vi "Write Service.vi"(8 "error in (no error)":errorcluster, 10 "Service":string, 11 "AWS Core in":refnum<class "NI_AWS_Core.lvclass">) -> (0 "error out":errorcluster, 3 "AWS Core out":refnum<class "NI_AWS_Core.lvclass">)   [LabVIEW 2015, in "NI_AWS_Core.lvclass"]
uses:
  NI_AWS_Core.lvclass
  NI_AWS_Core.lvclass/NI_AWS_Core.ctl
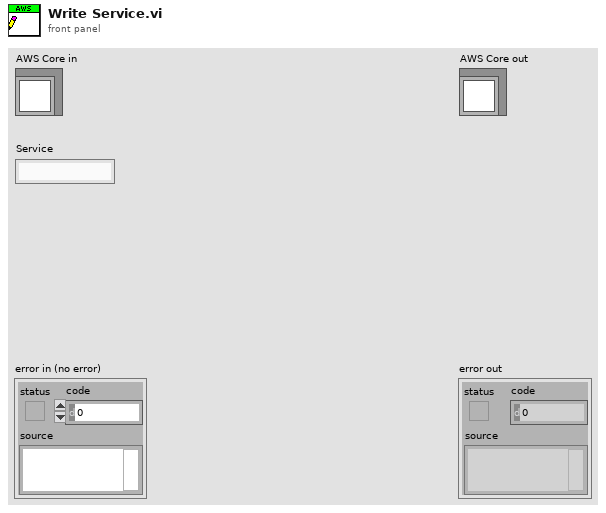
[diagram p1: front panel]
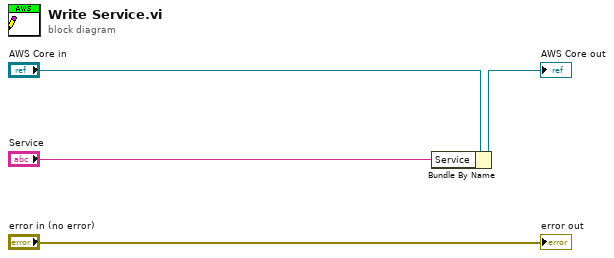
[diagram p0: block diagram]
diagram:
  n1 = Bundle By Name(cluster="AWS Core in", "Service"="Service") -> (→"AWS Core out":refnum<class "NI_AWS_Core.lvclass">)
  "error out" <- "error in (no error)"
